vi "Agilent 681x Acquire Power Measurement_eventCase.vi"() -> ()   [LabVIEW 2019]
doc: "Shows how to acquire a power measurement using low level data VIs."
uses:
  <vilib>/Utility/error.llb/DialogType.ctl
  <instrlib>/Agilent 681x Series/Public/Data/Low Level/Fetch Single Measurement (Power).vi
  <instrlib>/Agilent 681x Series/Agilent 681x Series.lvlib
panel:
  in  "Sample Spacing (25 us)":dbl=2.5e-05 format="%^.2g"
  in  "Sense Source (0: Internal)":u16(ring) items=["Internal", "External"]
  in  "Output Frequency (60 Hz)":dbl=60.0 format="%#.4g"
  in  "Voltage Amplitude (1.0 V)":dbl=1.0 format="%#.4g"
  in  "Relative Trigger Samples (0)":i32
  in  "Output Waveform Type (0: Sinusoid)":u16(ring) items=["Sinusoid", "Square", "Clipped Sinusoid", "User Specified"]
  out "Total Power":dbl
  out "Power Factor":dbl
  out "Reactive Power":dbl
  out "Apparent Power":dbl
  out "Real Power":dbl
  out "DC Power":dbl
  in  "Maximum Time (10000 ms)":i32=10000
  in  "User-Specified Output Waveform Name":string
  in  "Serial Configuration":T1={"Baud Rate"=9600, "Parity"=0, "Data Bits"=8} {"Data Bits" items=["7"=7, "8"=8]; "Parity" items=["None", "Odd", "Even", "Mark", "Space"]; "Baud Rate" items=["300"=300, "600"=600, "1200"=1200, "2400"=2400, "4800"=4800, "9600"=9600]}
  in  "VISA resource name":refnum<visa-resource-name>
  # "(c) 2008-2021 National Instruments Corp.  ALL RIGHTS RESERVED."
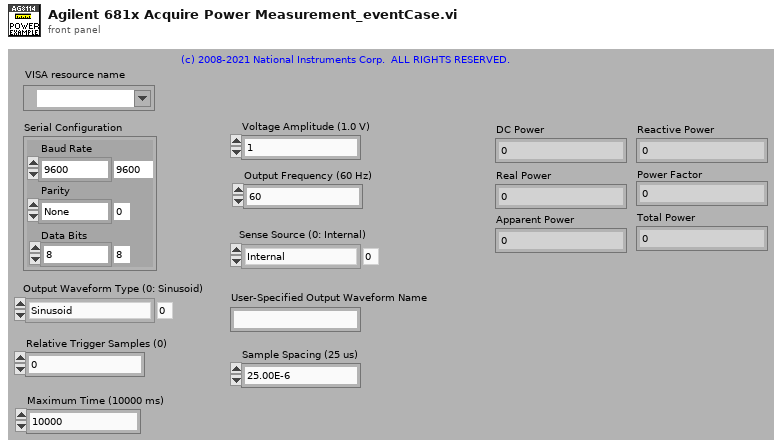
[diagram p1: front panel]
types:
  T1 = cluster{"Baud Rate":u32, "Parity":u16, "Data Bits":u16}
  T2 = typedef "DialogType.ctl" = u16
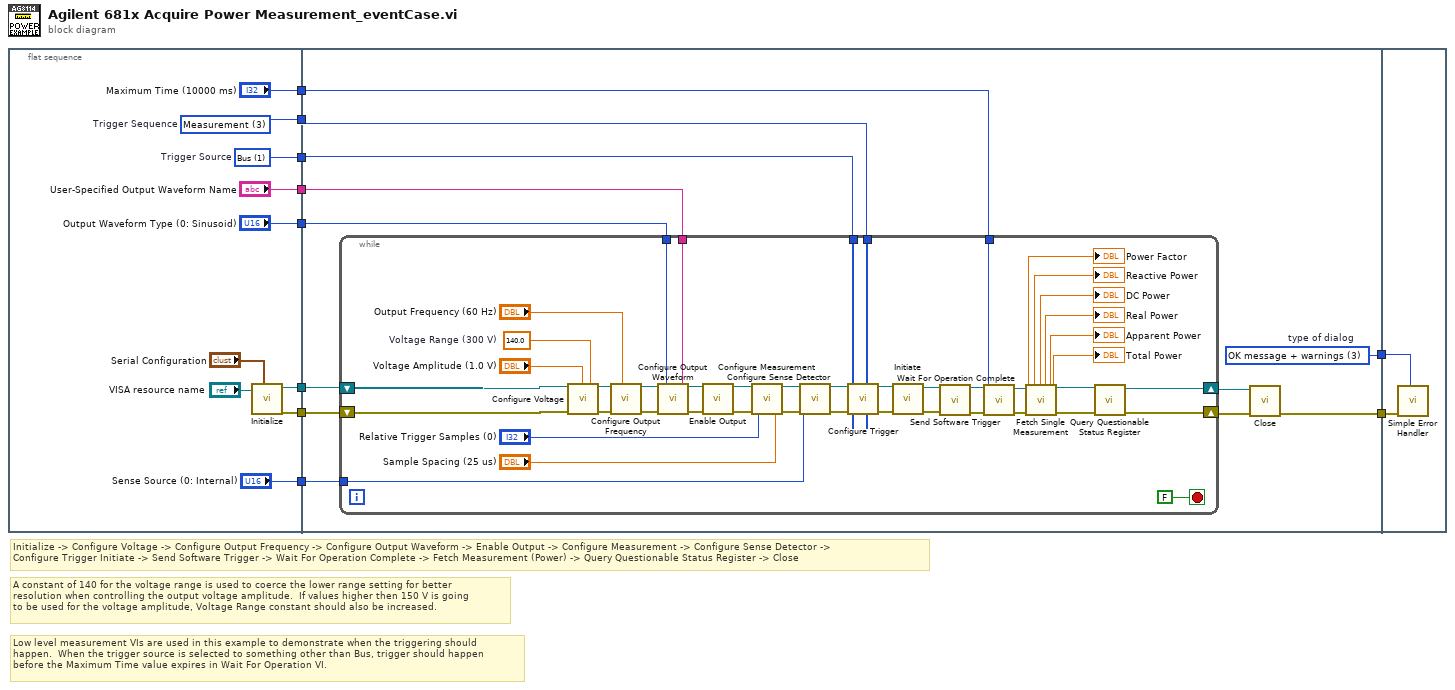
[diagram p0: block diagram]
diagram:
  # "Low level measurement VIs are used in this example to demonstrate when the triggering should\nhappen.  When the trigger source is selected to something other than Bus, trigger should happen\nbefore the Maximum Time value expires in Wait For Operation VI."
  # "A constant of 140 for the voltage range is used to coerce the lower range setting for better\nresolution when controlling the output voltage amplitude.  If values higher then 150 V is going\nto be used for the voltage amplitude, Voltage Range constant should also be increased."
  # "Initialize -> Configure Voltage -> Configure Output Frequency -> Configure Output Waveform -> Enable Output -> Configure Measurement -> Configure Sense Detector -> \nConfigure Trigger Initiate -> Send Software Trigger -> Wait For Operation Complete -> Fetch Measurement (Power) -> Query Questionable Status Register -> Close"
  n1 = flat-sequence {
    tunnel: ["Maximum Time (10000 ms)"] -> w10
    tunnel: [w17] -> w9
    tunnel: [w16] -> w8
    tunnel: ["Sense Source (0: Internal)"] -> w7
    tunnel: ["User-Specified Output Waveform Name"] -> w6
    tunnel: ["Output Waveform Type (0: Sinusoid)"] -> w5
    tunnel: [w12] -> w4
    tunnel: [w11] -> w3
    tunnel: w10 -> [w30]
    tunnel: w9 -> [w29]
    tunnel: w8 -> [w28]
    tunnel: w7 -> [w27]
    tunnel: w6 -> [w26]
    tunnel: w5 -> [w25]
    tunnel: w4 -> [w24]
    tunnel: w3 -> [w23]
    tunnel: [w22] -> w2
    tunnel: [w21] -> w1
    tunnel: w2 -> [w78]
    tunnel: w1 -> [w77]
    frame #0 {
      w16 = 1 items=["Immediate", "Bus", "External", "Phase", "Trigger Out"]  # Trigger Source
      w17 = 3 items=["Output"=1, "Synchronous Source"=2, "Measurement"=3]  # Trigger Sequence
      n2 = call <instrlib>:"Initialize.vi"("Serial Configuration"="Serial Configuration", "VISA resource name"="VISA resource name") -> ("error out"=w11:errorcluster, "VISA resource name out"=w12:refnum<visa-resource-name>)  [unwired: 8 in]
    }
    frame #1 {
      w22 = T2 3 items=["no dialog", "OK message", "continue or stop message", "OK message + warnings", "continue/stop + warnings"]  # type of dialog
      n3 = while {
        tunnel: w30 -> [w52]
        tunnel: w29 -> [w51]
        tunnel: w28 -> [w50]
        tunnel: w27 -> [w49]
        tunnel: w26 -> [w48]
        tunnel: w25 -> [w47]
        shift-right: [w76] -> w32
        shift-left: w24 -> [w46]
        shift-right: [w75] -> w31
        shift-left: w23 -> [w45]
        stop <- FALSE stop-if-true
        w42 = 140.0  # Voltage Range (300 V)
        n4 = call <instrlib>:"Configure Voltage.vi"("VISA resource name"=w46, "Voltage Range (300 V)"=w42, "Voltage Amplitude (1.0 V)"="Voltage Amplitude (1.0 V)", "error in (no error)"=w45) -> ("VISA resource name out"=w62:refnum<visa-resource-name>, "error out"=w61:errorcluster)  [unwired: 10 in]
        n5 = call <instrlib>:"Configure Output Frequency.vi"("VISA resource name"=w62, "Output Frequency (60 Hz)"="Output Frequency (60 Hz)", "error in (no error)"=w61) -> ("VISA resource name out"=w56:refnum<visa-resource-name>, "error out"=w55:errorcluster)  [unwired: 11 in]
        n6 = call <instrlib>:"Configure Output Waveform.vi"("VISA resource name"=w56, "User-Specified Output Waveform Name"=w48, "Output Waveform Type (0: Sinusoid)"=w47, "error in (no error)"=w55) -> ("VISA resource name out"=w54:refnum<visa-resource-name>, "error out"=w53:errorcluster)  [unwired: 10 in]
        n7 = call <instrlib>:"Enable Output.vi"("VISA resource name"=w54, "error in (no error)"=w53) -> ("VISA resource name out"=w57:refnum<visa-resource-name>, "error out"=w58:errorcluster)  [unwired: 12 in]
        n8 = call <instrlib>:"Configure Measurement.vi"("VISA resource name"=w57, "Relative Trigger Samples (0)"="Relative Trigger Samples (0)", "Sample Spacing (25 us)"="Sample Spacing (25 us)", "error in (no error)"=w58) -> ("VISA resource name out"=w59:refnum<visa-resource-name>, "error out"=w60:errorcluster)  [unwired: 10 in]
        n9 = call <instrlib>:"Configure Sense Detector.vi"("VISA resource name"=w59, "Sense Source (0: Internal)"=w49, "error in (no error)"=w60) -> ("VISA resource name out"=w64:refnum<visa-resource-name>, "error out"=w63:errorcluster)  [unwired: 11 in]
        n10 = call <instrlib>:"Configure Trigger.vi"("VISA resource name"=w64, "Trigger Sequence (1: Output 1)"=w51, "Trigger Source (0: Immediate)"=w50, "error in (no error)"=w63) -> ("VISA resource name out"=w66:refnum<visa-resource-name>, "error out"=w65:errorcluster)  [unwired: 10 in]
        n11 = call <instrlib>:"Initiate.vi"("error in (no error)"=w65, "VISA resource name"=w66) -> ("error out"=w68:errorcluster, "VISA resource name out"=w67:refnum<visa-resource-name>)  [unwired: 8 in]
        n12 = call <instrlib>:"Send Software Trigger.vi"("VISA resource name"=w67, "error in (no error)"=w68) -> ("VISA resource name out"=w70:refnum<visa-resource-name>, "error out"=w69:errorcluster)  [unwired: 12 in]
        n13 = call <instrlib>:"Wait For Operation Complete.vi"("error in (no error)"=w69, "Maximum Time (10000 ms)"=w52, "VISA resource name"=w70) -> ("error out"=w72:errorcluster, "VISA resource name out"=w71:refnum<visa-resource-name>)  [unwired: 7 in]
        n14 = call-poly <instrlib>:"Fetch Single Measurement.vi"("VISA resource name"=w71, "error in (no error)"=w72) -> ("Power Factor"=→"Power Factor":dbl, "Reactive Power"=→"Reactive Power":dbl, "VISA resource name out"=w74:refnum<visa-resource-name>, "DC Power"=→"DC Power":dbl, "Real Power"=→"Real Power":dbl, "Apparent Power"=→"Apparent Power":dbl, "Total Power"=→"Total Power":dbl, "error out"=w73:errorcluster)  [unwired: 6 in]
        n15 = call <instrlib>:"Query Questionable Status Register.vi"("error in (no error)"=w73, "VISA resource name"=w74) -> ("error out"=w75:errorcluster, "VISA resource name out"=w76:refnum<visa-resource-name>)  [unwired: 7 in, 1 out]
      }
      n16 = call <instrlib>:"Close.vi"("error in (no error)"=w31, "VISA resource name"=w32) -> ("error out"=w21:errorcluster)  [unwired: 9 in]
    }
    frame #2 {
      n17 = call <vilib>:"Simple Error Handler.vi"("type of dialog (OK msg:1)"=w78, "error in (no error)"=w77) -> ()  [unwired: 3 in, 5 out]
    }
  }
